vi "SubVI ATI.vi"() -> ()   [LabVIEW 2011]
uses:
  GLOBAL -MAIN.vi
  ctlSeqFNs_SubVI PhaseSpace.ctl
  ctlSeqFNs_SubVI ATI.ctl
  NCML-PhaseSpace/ctrOWLMarker.ctl
  C:/Program Files/Phasespace/libowlsock.dll
  NCML-PhaseSpace/ctrSetsFlags.ctl
  NCML-PhaseSpace/ctrCommonFlags.ctl
  ctlPkgATI.ctl
  <vilib>/Analysis/Matrix/Datatypes/RealMatrix.ctl
  <vilib>/Analysis/Matrix/NI_Matrix.lvlib
panel:
  out "markers obtained (err: <0)":u16
  out "markers":T1[](array[typedef])
  in  "marker count":i32=16
  out "connected?":bool
  in  "server IP":string="192.168.0.101"
  in  "STOP":bool
  # "Parallel SubVI ATI"
  # "Acquires PhaseSpace data and Trigger signal\nSaves TDMS file."
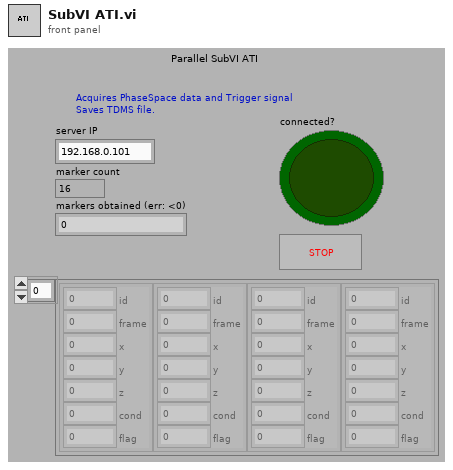
[diagram p1: front panel]
types:
  T1 = typedef "ctrOWLMarker.ctl" = cluster{"id":i32, "frame":i32, "x":sgl, "y":sgl, "z":sgl, "cond":sgl, "flag":u32}
  T2 = typedef "ctlPkgATI.ctl" = cluster{"VIRef":refnum<vi>, "ATI":refnum<k34>, "ATI1 Ch names":string[], "tick ini":i64, "PhaseSpace":refnum<queue>, "Trigger array":u8[], "connected to server?":bool, "ATI2 Ch names":string[], "ATI3 Ch names":string[], "ATI4 Ch names":string[], "DAQmx1":refnum<k21>, "DAQmx2":refnum<k21>, "DAQmx3":refnum<k21>, "DAQmx4":refnum<k21>, "CalibMatrix1":T3, "CalibMatrix2":T3, "CalibMatrix3":T3, "CalibMatrix4":T3}
  T3 = typedef "NI_Matrix.lvlib/RealMatrix.ctl" = dbl[][]
  T4 = typedef "ctlSeqFNs_SubVI PhaseSpace.ctl" = enum16{"INITIALIZE", "IDLE", "READY", "SEND2MAIN", "TRIGGER", "END", "ERROR", "EXIT"}
  T5 = enum16{"open", "open or create", "create or replace", "create", "open (read-only)"}
  T6 = typedef "ctlSeqFNs_SubVI ATI.ctl" = enum16{"INITIALIZE", "IDLE", "READY", "START", "HOLD", "Convert deg F to deg C", "Send to Main", "Main Event Msg", "ERROR", "EXIT"}
  T7 = enum16{"ALIGN -CENTER", "ALIGN -TOP LEFT", "ALIGN -AS IS", "ALIGN -CUSTOM"}
  T8 = typedef "ctrCommonFlags.ctl" = u16
  T9 = typedef "ctrSetsFlags.ctl" = u16
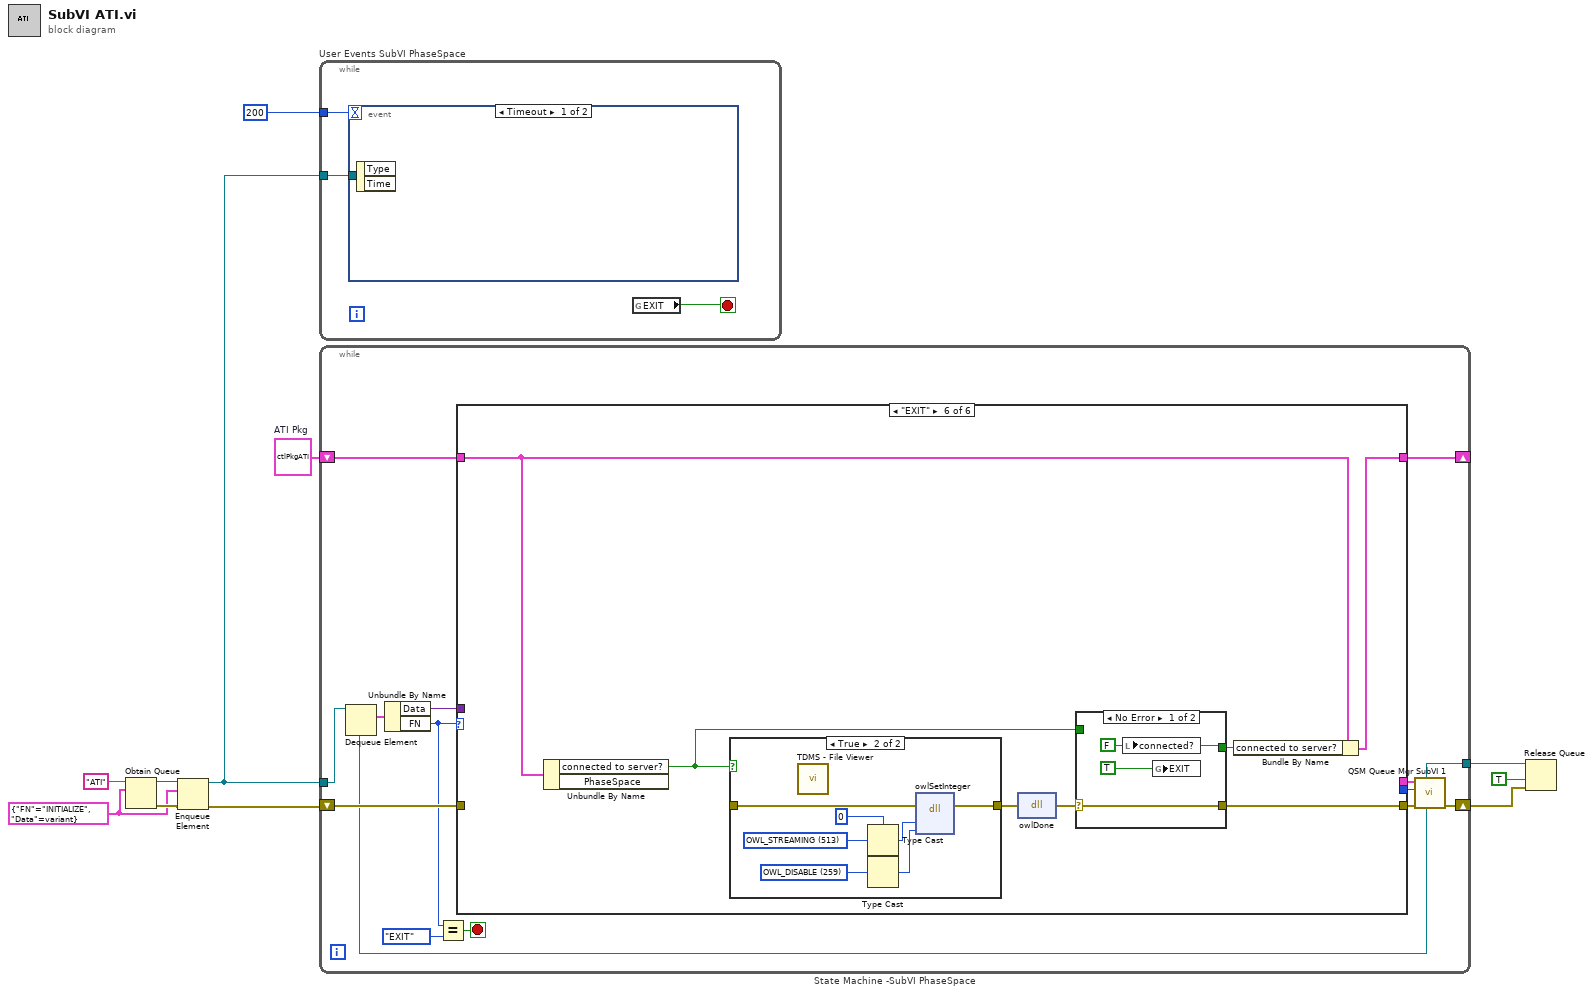
[diagram p0: block diagram]
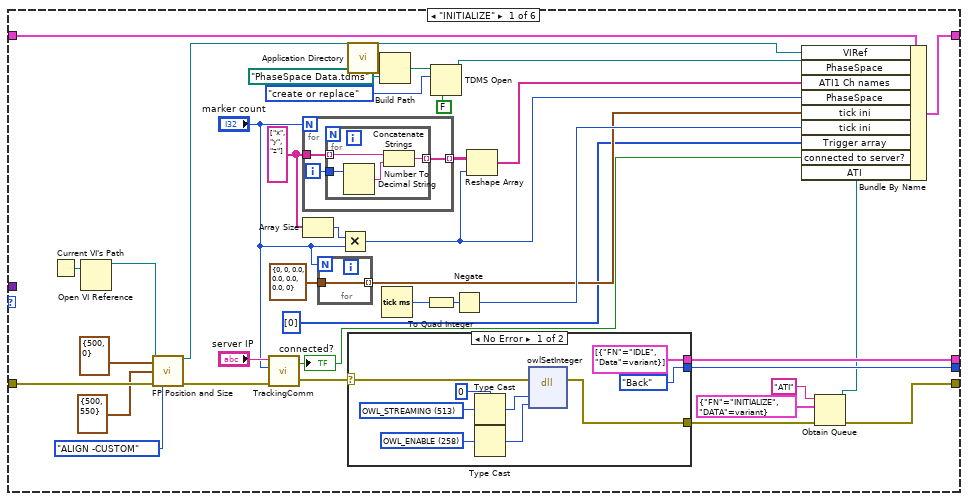
[diagram p2: hidden frame]
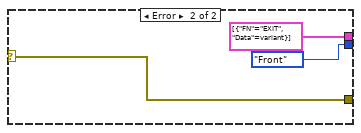
[diagram p3: hidden frame]
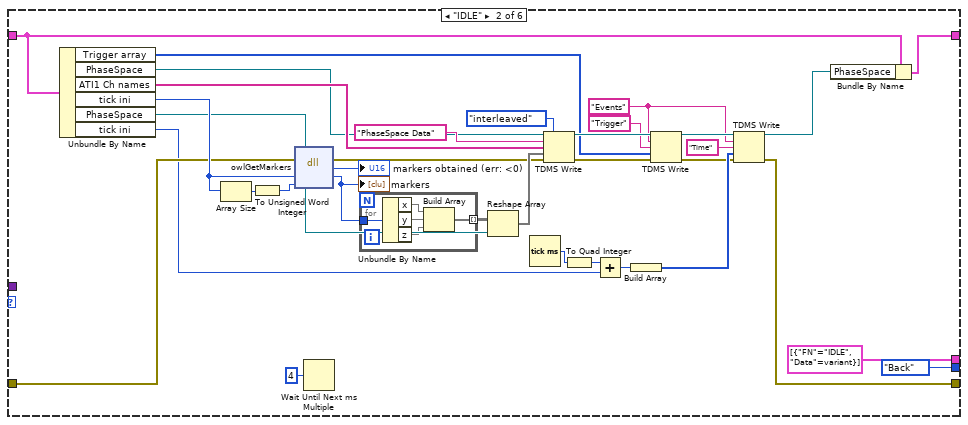
[diagram p4: hidden frame]
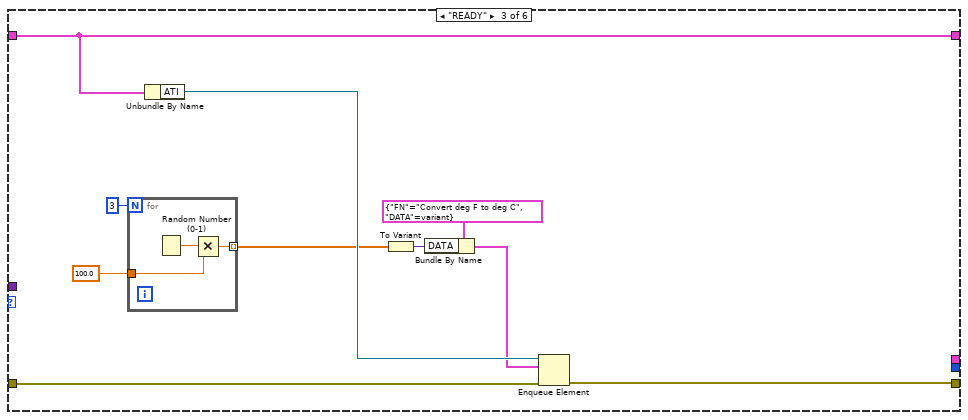
[diagram p5: hidden frame]
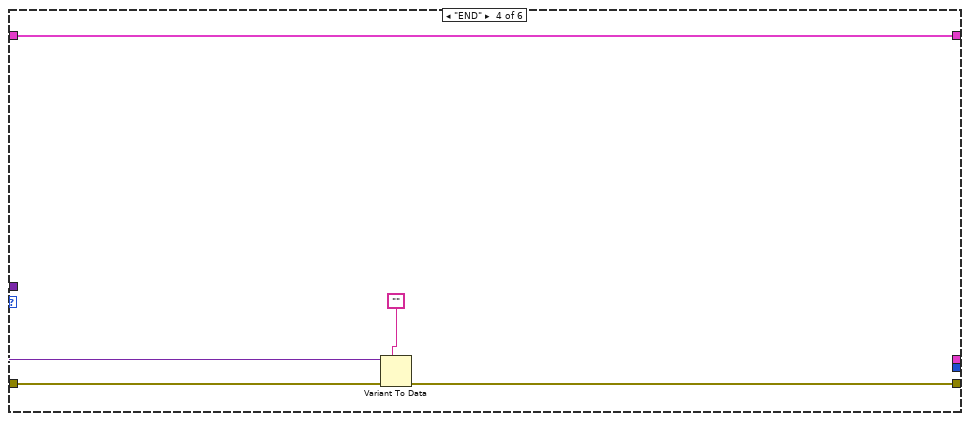
[diagram p6: hidden frame]
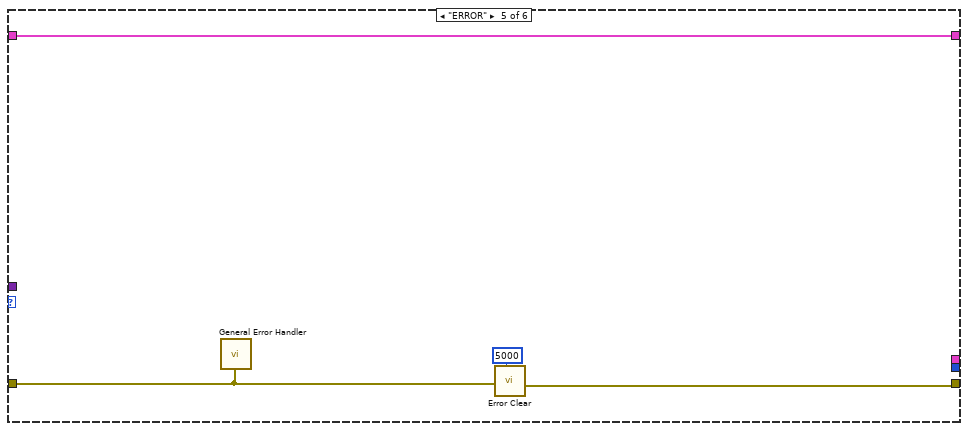
[diagram p7: hidden frame]
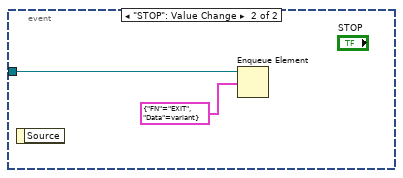
[diagram p10: hidden frame]
diagram:
  w2 = T2 {"VIRef"=refnum, "ATI"=refnum, "ATI1 Ch names"=[], "tick ini"=0, "PhaseSpace"=refnum, "Trigger array"=[], "connected to server?"=FALSE, "ATI2 Ch names"=[], "ATI3 Ch names"=[], "ATI4 Ch names"=[], "DAQmx1"="", "DAQmx2"="", "DAQmx3"="", "DAQmx4"="", "CalibMatrix1"=[], "CalibMatrix2"=[], "CalibMatrix3"=[], "CalibMatrix4"=[]}  # ATI Pkg
  w6 = cluster{"FN":T4, "Data":variant} {"FN"=enum."INITIALIZE", "Data"=variant} ("cluFNData")
  n1 = Obtain Queue(name (unnamed)="ATI", element data type=w6) -> (queue out=w7:refnum<queue>, error out=w9:errorcluster)  [unwired: 3 in, 1 out]
  n2 = Enqueue Element(queue=w7, element=w6, error in (no error)=w9) -> (queue out=w3:refnum<queue>, error out=w8:errorcluster)  [unwired: 1 in, 1 out]
  n3 = while "User Events SubVI PhaseSpace" {
    tunnel: 200 -> [w14]
    tunnel: w3 -> [w12]
    stop <- w13 stop-if-true
    n4 = event shown="[0] Timeout" {
      selector: _ -> [_ _]
      dyn-events: _ -> [_ _]
      timeout: w14 -> [_ _]
      tunnel: w12 -> [_ w16]
      event Timeout {
        n5 = event-data() -> ()  [unwired: 1 in, 2 out]
      }
      event "STOP": Value Change {
        n6 = event-data() -> ()  [unwired: 1 in, 1 out]
        n7 = Enqueue Element(queue=w16, element=cluster{"FN":T4, "Data":variant} {"FN"=enum."EXIT", "Data"=variant}) -> ()  [unwired: 2 in, 3 out]
      }
    }
    n8 = global read "GLOBAL -MAIN.vi" "EXIT"() -> (w13:bool)
  }
  n9 = while "State Machine -SubVI PhaseSpace" {
    shift-right: [w20] -> w1
    shift-left: w8 -> [w30]
    tunnel: w3 -> [w27]
    tunnel: [w17] -> w5
    shift-right: [w22] -> _
    shift-left: w2 -> [w23]
    stop <- w29 stop-if-true
    n10 = Dequeue Element(queue=w27) -> (queue out=w17:refnum<queue>, element=w26:cluster{"FN":T4, "Data":variant})  [unwired: 2 in, 2 out]
    n11 = Unbundle By Name(w26) -> ("Data"=w25:variant, "FN"=w24:T4)
    n12 = Equal?(x=w24, y=ctlSeqFNs_SubVI_PhaseSpace."EXIT" ("FN")) -> (x = y?=w29:bool)
    n13 = case shown="\"EXIT\"" w24 {
      tunnel: w30 -> [w66 w104 w137 w142 w146 w157]
      tunnel: [w61 w98 w136 w141 w148 w150] -> w21
      tunnel: w25 -> [_ _ _ w144 _ _]
      tunnel: w23 -> [w47 w101 w128 w145 w149 w155]
      tunnel: [w65 w99 w128 w145 w149 w154] -> w22
      tunnel: [w35 cluster{"FN":T4, "Data":variant}[] [{"FN"=enum."IDLE", "Data"=variant}] ("QFNs") _ _ _ _] -> w18
      tunnel: [w34 enum16{"Back", "Front", "Replace"}."Back" ("Enum") _ _ _ _] -> w19
      frame "INITIALIZE" {
        w48 = string[] ["x", "y", "z"]
        n14 = Current VI's Path() -> (path=w68:path)
        n15 = Open VI Reference(vi path=w68) -> (vi reference=w67:refnum<vi>)  [unwired: 5 in, 1 out]
        n16 = call "FP Position and Size.vi"("VIRefNum  IN"=w67, "Poistion"=cluster{"left":i16, "top":i16} {"left"=500, "top"=0}, "Size"=cluster{"right":i16, "bottom":i16} {"right"=500, "bottom"=550}, "error in (no error)"=w66, "Mode"=T7."ALIGN -CUSTOM") -> ("VIRefNum OUT"=w33:refnum<vi>, "error out"=w55:errorcluster)  [unwired: 9 in]
        n17 = call "TrackingComm.vi"("error in (no error)"=w55, "marker tally (default: 32)"="marker count", "server address"="server IP") -> ("error out"=w56:errorcluster, "connected to server?"=w31:bool)  [unwired: 1 in]
        "connected?" <- w31
        n18 = for {
          N: "marker count" -> [_]
          tunnel: w48 -> [w71]
          tunnel: [w69] -> w53 mode=indexing
          i -> [w70]
          n19 = for {
            tunnel: w71 -> [w75] mode=indexing
            tunnel: w70 -> [w74]
            tunnel: [w72] -> w69 mode=indexing
            n20 = Number To Decimal String(number=w74) -> (decimal integer string=w73:string)  [unwired: 1 in]
            n21 = Concatenate Strings(w75, w73) -> (w72:string)
          }
        }
        n22 = Array Size(array=w48) -> (size(s)=w49:i32)
        n23 = for {
          N: "marker count" -> [_]
          tunnel: T1 {"id"=0, "frame"=0, "x"=0.0, "y"=0.0, "z"=0.0, "cond"=0.0, "flag"=0} -> [w88]
          tunnel: [w88] -> w44 mode=indexing
        }
        n24 = Multiply(x=w49, y="marker count") -> (x*y=w43:i32)
        n25 = call <vilib>:"Application Directory.vi"() -> ("Application Directory"=w39:path)
        n26 = case shown="No Error" w56 {
          selector: w56 -> [w79 w87]
          tunnel: [w78 w87] -> w54
          tunnel: [cluster{"FN":T4, "Data":variant}[] [{"FN"=enum."IDLE", "Data"=variant}] ("QFNs") cluster{"FN":T4, "Data":variant}[] [{"FN"=enum."EXIT", "Data"=variant}] ("QFNs")] -> w35
          tunnel: [enum16{"Back", "Front", "Replace"}."Back" ("Enum") enum16{"Back", "Front", "Replace"}."Front" ("Enum")] -> w34
          frame No Error {
            w84 = u16 0
            w81 = T8 258 items=["OWL_CREATE"=256, "OWL_DESTROY"=257, "OWL_ENABLE"=258, "OWL_DISABLE"=259] ("Common flages")
            w80 = T9 513 items=["OWL_FREQUENCY"=512, "OWL_STREAMING"=513, "OWL_INTERPOLATION"=514, "OWL_BUTTONS"=528, "OWL_MARKERS"=529, "OWL_RIGIDS"=530, "OWL_COMMDATA"=544, "OWL_TIMESTAMP"=545, "OWL_PLANES"=672, "OWL_DETECTORS"=673, "OWL_IMAGES"=674, "OWL_TRANSFORM"=49664] ("Sets flags")
            n27 = Type Cast(type=w84, x=w80) -> (*(type *) &x=w83:u16)
            n28 = Type Cast(type=w84, x=w81) -> (*(type *) &x=w82:u16)
            n29 = dll-call lib="C:/Program Files/Phasespace/libowlsock.dll" fn="owlSetInteger"(error in=w79, "pname"=w83, "param"=w82) -> (error out=w78:errorcluster)  [unwired: 4 in, 2 out]
          }
          frame Error {
          }
        }
        n30 = Build Path(base path=w39, name or relative path=path "PhaseSpace Data.tdms" ("file path")) -> (appended path=w38:path)
        n31 = Tick Count (ms)() -> (millisecond timer value=w51:u32)
        n32 = To Quad Integer(1:w51) -> (0:w52:i64)
        n33 = TDMS Open(6:FALSE ("disable buffering? (T)"), 10:T5."create or replace" ("operation"), 11:w38) -> (3:w37:refnum<k34>)  [unwired: 3 in, 1 out]
        n34 = Negate(x=w52) -> (-x=w46:i64)
        n35 = Reshape Array(w53, w43) -> (w45:string[])
        n36 = Obtain Queue(name (unnamed)="ATI", element data type=cluster{"FN":T6, "DATA":variant} {"FN"=enum."INITIALIZE", "DATA"=variant} ("cluFNData"), error in (no error)=w54) -> (queue out=w32:refnum<queue>, error out=w61:errorcluster)  [unwired: 2 in, 1 out]
        n37 = Bundle By Name(cluster=w47, "VIRef"=w33, "PhaseSpace"=w37, "ATI1 Ch names"=w45, "PhaseSpace"=w43, "tick ini"=w44, "tick ini"=w46, "Trigger array"=u8[] [0], "connected to server?"=w31, "ATI"=w32) -> (w65:T2)
      }
      frame "IDLE" {
        w91 = "Events" ("group name")
        n38 = Unbundle By Name(w101) -> ("Trigger array"=w89:u8[], "PhaseSpace"=w111:refnum<queue>, "ATI1 Ch names"=w112:string[], "tick ini"=w116:i64, "PhaseSpace"=w115:refnum<queue>, "tick ini"=w102:i64)
        n39 = Array Size(array=w116) -> (size(s)=w120:i32)
        n40 = To Unsigned Word Integer(number=w120) -> (unsigned 16bit integer=w121:u16)
        n41 = dll-call lib="C:/Program Files/Phasespace/libowlsock.dll" fn="owlGetMarkers"(error in=w104, "markers"=w116, "count"=w121) -> (error out=w109:errorcluster, "return type"=→"markers obtained (err: <0)":u16, "markers"=w117:i64)  [unwired: 3 in, 1 out]
        "markers" <- w117
        n42 = Wait Until Next ms Multiple(millisecond multiple=u32 4) -> ()  [unwired: 1 out]
        n43 = for {
          tunnel: w117 -> [w127]
          tunnel: [w123] -> w118 mode=indexing
          n44 = Unbundle By Name(w127) -> ("x"=w126, "y"=w125, "z"=w124)
          n45 = Build Array(w126, w125, w124) -> (w123:void[])
        }
        n46 = Reshape Array(w118, w115) -> (w110:void[])
        n47 = Tick Count (ms)() -> (millisecond timer value=w107:u32)
        n48 = TDMS Write(0:w111, 1:enum16{"decimated", "interleaved"}."interleaved" ("data layout (0:decimated)"), 5:"PhaseSpace Data" ("group name"), 7:w112, 9:w110, 11:w109) -> (4:w95:refnum<k34>, 15:w94:errorcluster)  [unwired: 2 out]
        n49 = To Quad Integer(1:w107) -> (0:w103:i64)
        n50 = Add(x=w103, y=w102) -> (x+y=w106:i64)
        n51 = Build Array(w106) -> (w105:i64[])
        n52 = TDMS Write(0:w95, 5:w91, 7:"Trigger" ("channel name"), 9:w89, 11:w94) -> (4:w92:refnum<k34>, 15:w93:errorcluster)  [unwired: 1 in, 2 out]
        n53 = TDMS Write(0:w92, 5:w91, 7:"Time" ("channel name"), 9:w105, 11:w93) -> (4:w100:refnum<k34>, 15:w98:errorcluster)  [unwired: 1 in, 2 out]
        n54 = Bundle By Name(cluster=w101, "PhaseSpace"=w100) -> (w99:T2)
      }
      frame "READY" {
        n55 = for {
          N: 3 -> [_]
          tunnel: [w139] -> w129 mode=indexing
          tunnel: 100.0 ("y") -> [w138]
          n56 = Random Number (0-1)() -> (number: 0 to 1=w140:dbl)
          n57 = Multiply(x=w140, y=w138) -> (x*y=w139:dbl)
        }
        n58 = Unbundle By Name(w128) -> ("ATI"=w135:refnum<k34>)
        n59 = To Variant(anything=w129) -> (Variant=w133:variant)
        n60 = Bundle By Name(cluster=cluster{"FN":T6, "DATA":variant} {"FN"=enum."Convert deg F to deg C", "DATA"=variant} ("element"), "DATA"=w133) -> (w132:cluster{"FN":T6, "DATA":variant})
        n61 = Enqueue Element(queue=w135, element=w132, error in (no error)=w137) -> (error out=w136:errorcluster)  [unwired: 1 in, 2 out]
      }
      frame "END" {
        n62 = Variant To Data(error in=w142, type="", Variant=w144) -> (error out=w141:errorcluster)  [unwired: 1 out]
      }
      frame "ERROR" {
        n63 = call <vilib>:"General Error Handler.vi"("error in (no error)"=w146) -> ()  [unwired: 10 in, 5 out]
        n64 = call "Error Clear.vi"("wait(ms)"=u32 5000, "error in"=w146) -> ("error in (no error)"=w148:errorcluster)  [unwired: 6 in]
      }
      frame "EXIT" {
        n65 = Unbundle By Name(w155) -> ("connected to server?"=w151:bool)  [unwired: 1 out]
        n66 = case shown="True" w151 {
          tunnel: _ -> [w163 w166]
          tunnel: [w163 w165] -> w156
          frame False {
          }
          frame True {
            w169 = u16 0
            w168 = T8 259 items=["OWL_CREATE"=256, "OWL_DESTROY"=257, "OWL_ENABLE"=258, "OWL_DISABLE"=259] ("Common flages")
            w167 = T9 513 items=["OWL_FREQUENCY"=512, "OWL_STREAMING"=513, "OWL_INTERPOLATION"=514, "OWL_BUTTONS"=528, "OWL_MARKERS"=529, "OWL_RIGIDS"=530, "OWL_COMMDATA"=544, "OWL_TIMESTAMP"=545, "OWL_PLANES"=672, "OWL_DETECTORS"=673, "OWL_IMAGES"=674, "OWL_TRANSFORM"=49664] ("Sets flags")
            n67 = call <vilib>:"TDMS - File Viewer.vi"() -> ("file path"=w164:path)  [unwired: 5 in, 2 out]
            n68 = Type Cast(type=w169, x=w167) -> (*(type *) &x=w170:u16)
            n69 = Type Cast(type=w169, x=w168) -> (*(type *) &x=w171:u16)
            n70 = dll-call lib="C:/Program Files/Phasespace/libowlsock.dll" fn="owlSetInteger"(error in=w166, "pname"=w170, "param"=w171) -> (error out=w165:errorcluster)  [unwired: 4 in, 2 out]
          }
        }
        n71 = dll-call lib="C:/Program Files/Phasespace/libowlsock.dll" fn="owlDone"(error in=w156) -> (error out=w153:errorcluster)  [unwired: 2 in, 2 out]
        n72 = case shown="No Error" w153 {
          selector: w153 -> [w158 w161]
          tunnel: [w160 w162] -> w152
          tunnel: w151 -> [_ w162]
          tunnel: [w158 w161] -> w150
          frame No Error {
            w160 = FALSE ("connected to server?")
            n73 = local write "connected?"(w160) -> ()
            n74 = global write "GLOBAL -MAIN.vi" "EXIT"(TRUE ("EXIT")) -> ()
          }
          frame Error {
          }
        }
        n75 = Bundle By Name(cluster=w155, "connected to server?"=w152) -> (w154:T2)
      }
    }
    n76 = call "QSM Queue Mgr SubVI 1.vi"("QRef"=w17, "Error IN"=w21, "FNs"=w19, "QSTATES"=w18) -> ("Error OUT"=w20:errorcluster)  [unwired: 4 in]
  }
  n77 = Release Queue(queue=w5, force destroy? (F)=TRUE, error in (no error)=w1) -> ()  [unwired: 3 out]
